vi "write_DAC_word.vi"(7 "converter box version":i16=1 min=1 max=2, 10 "U16 data number":u16, 11 "DAC values in":T1={"DAC channel enable"={"ch0"=TRUE, "ch1"=TRUE, "ch2"=TRUE, "ch3"=TRUE, "ch4"=TRUE, "ch5"=TRUE, "ch6"=TRUE}, "DAC voltage"={"ch0"=0, "ch1"=0, "ch2"=0, "ch3"=0, "ch4"=0, "ch5"=0, "ch6"=0}, "offset"=0, "channel index"=0, "bit index"=0, "synch?"=FALSE, "DAC clock"=FALSE, "finished?"=FALSE} {"bit index" min=-1 max=17 step=1; "channel index" max=7 step=1; "offset" max=4095; "DAC voltage"."ch6" max=4095 step=1; "DAC voltage"."ch5" max=4095 step=1; "DAC voltage"."ch4" max=4095 step=1; "DAC voltage"."ch3" max=4095 step=1; "DAC voltage"."ch2" max=4095 step=1; "DAC voltage"."ch1" max=4095 step=1; "DAC voltage"."ch0" max=4095 step=1}) -> (3 "DAC values out":T1={"DAC channel enable"={"ch0"=TRUE, "ch1"=TRUE, "ch2"=TRUE, "ch3"=TRUE, "ch4"=TRUE, "ch5"=TRUE, "ch6"=TRUE}, "DAC voltage"={"ch0"=0, "ch1"=0, "ch2"=0, "ch3"=0, "ch4"=0, "ch5"=0, "ch6"=0}, "offset"=0, "channel index"=0, "bit index"=0, "synch?"=FALSE, "DAC clock"=FALSE, "finished?"=FALSE} {"bit index" min=-1 max=17 step=1; "channel index" max=7 step=1; "offset" max=4095; "DAC voltage"."ch6" max=4095 step=1; "DAC voltage"."ch5" max=4095 step=1; "DAC voltage"."ch4" max=4095 step=1; "DAC voltage"."ch3" max=4095 step=1; "DAC voltage"."ch2" max=4095 step=1; "DAC voltage"."ch1" max=4095 step=1; "DAC voltage"."ch0" max=4095 step=1})   [LabVIEW 2010]
uses:
  common_typedefs/DAC_values_cluster.ctl
  common_typedefs/DAC_channel_enable_cluster.ctl
  common_typedefs/DAC_voltage_cluster.ctl
  <vilib>/eio/EIONode/EIONode.xnode
  <vilib>/rvi/eio/nirviEIOImplementation/nirviEIOImplementation.xnode
  <vilib>/rvi/eio/common/nirviEmuClasses.ctl
  <vilib>/rvi/eio/common/nirviEmuTemplateMethod_noerrors.vi
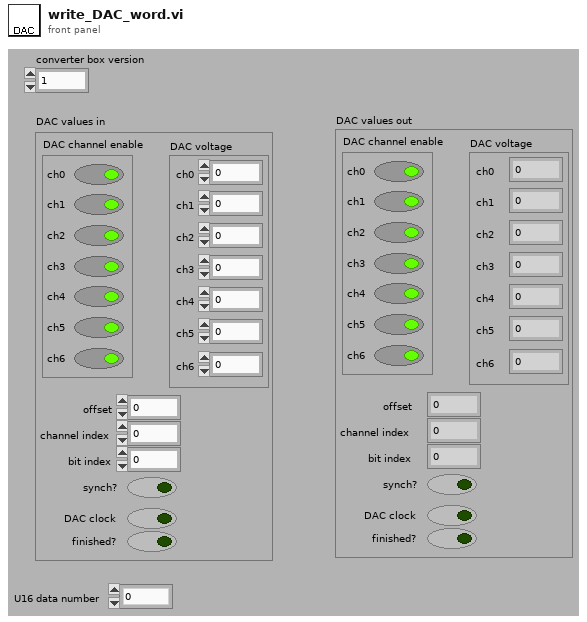
[diagram p1: front panel]
types:
  T1 = typedef "DAC_values_cluster.ctl" = cluster{"DAC channel enable":T2, "DAC voltage":T3, "offset":u16, "channel index":u16, "bit index":i32, "synch?":bool, "DAC clock":bool, "finished?":bool}
  T2 = typedef "DAC_channel_enable_cluster.ctl" = cluster{"ch0":bool, "ch1":bool, "ch2":bool, "ch3":bool, "ch4":bool, "ch5":bool, "ch6":bool}
  T3 = typedef "DAC_voltage_cluster.ctl" = cluster{"ch0":u16, "ch1":u16, "ch2":u16, "ch3":u16, "ch4":u16, "ch5":u16, "ch6":u16}
  T4 = typedef "nirviEmuClasses.ctl" = enum16{"IO Read", "IO Write", "Method", "Property Read", "Property Write"}
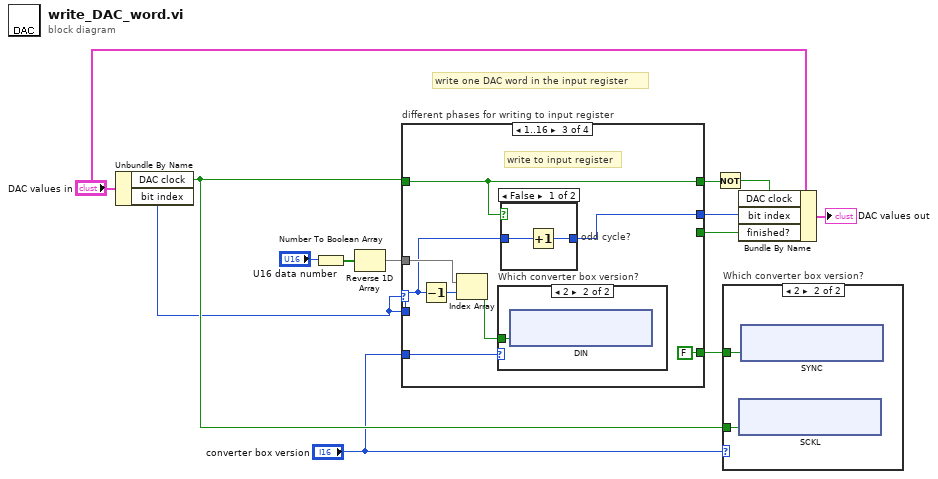
[diagram p0: block diagram]
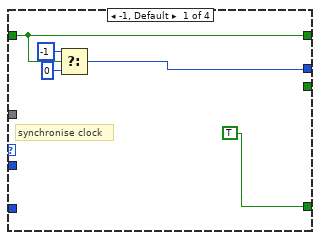
[diagram p3: hidden frame]
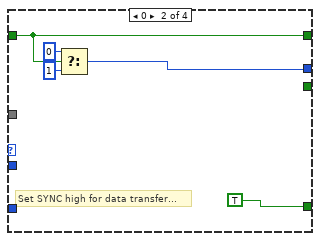
[diagram p4: hidden frame]
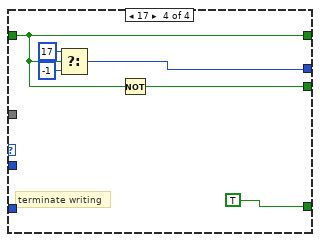
[diagram p7: hidden frame]
diagram:
  # "write one DAC word in the input register"
  n1 = Unbundle By Name("DAC values in") -> ("DAC clock"=w8:bool, "bit index"=w7:i32)
  n2 = Number To Boolean Array(number="U16 data number") -> (Boolean array=w13:bool[])
  n3 = Reverse 1D Array(array=w13) -> (reversed array=w11:bool[])
  n4 = case "different phases for writing to input register" shown="1..16" w7 {
    tunnel: w8 -> [w16 w19 w29 w48]
    tunnel: [w15 w21 w27 w50] -> w4
    tunnel: [TRUE ("SYNC") TRUE ("SYNC") FALSE ("SYNC") TRUE ("SYNC")] -> w9
    tunnel: w7 -> [_ _ w28 _]
    tunnel: w11 -> [_ _ w30 _]
    tunnel: [w16 w19 w29 w48] -> w10
    tunnel: [_ _ _ w47] -> w3
    tunnel: "converter box version" -> [_ _ w24 _]
    frame -1, Default {
      # "synchronise clock"
      n5 = Select(t=-1, s=w16, f=0) -> (s? t:f=w15:i32)
    }
    frame 0 {
      # "Set SYNC high for data transfer..."
      n6 = Select(t=0, s=w19, f=1) -> (s? t:f=w21:i32)
    }
    frame 1..16 {
      # "write to input register"
      n7 = Decrement(x=w28) -> (x-1=w31:i32)
      n8 = Index Array(array=w30, index=w31) -> (element=w25:bool)
      n9 = case "Which converter box version?" shown="2" w24 {
        tunnel: w25 -> [_ w32]
        frame Default {
        }
        frame 2 {
          n10 = xnode "DIN"("Connector1/DIO36"=w32) -> ()  [unwired: 1 in, 1 out]
        }
      }
      n11 = case "odd cycle?" shown="False" w29 {
        tunnel: w28 -> [w44 w46]
        tunnel: [w45 w46] -> w27
        frame False {
          n12 = Increment(x=w44) -> (x+1=w45:i32)
        }
        frame True {
        }
      }
    }
    frame 17 {
      # "terminate writing"
      n13 = Select(t=17, s=w48, f=-1) -> (s? t:f=w50:i32)
      n14 = Not(x=w48) -> (.not. x?=w47:bool)
    }
  }
  n15 = Not(x=w10) -> (.not. x?=w5:bool)
  n16 = case "Which converter box version?" shown="2" "converter box version" {
    tunnel: w9 -> [_ w54]
    tunnel: w8 -> [_ w53]
    frame Default {
    }
    frame 2 {
      n17 = xnode "SCKL"("Connector1/DIO38"=w53) -> ()  [unwired: 1 in, 1 out]
      n18 = xnode "SYNC"("Connector1/DIO34"=w54) -> ()  [unwired: 1 in, 1 out]
    }
  }
  n19 = Bundle By Name(cluster="DAC values in", "DAC clock"=w5, "bit index"=w4, "finished?"=w3) -> (→"DAC values out":T1)
